vi "ReadUarmCoordinatesCompareV3.vi"(6 "error in":errorcluster, 8 "Machine In":refnum<visa-resource-name>, 9 "INPUT Z Coord":dbl, 10 "INPUT X Coord":dbl, 11 "INPUT Y Coord":dbl) -> (0 "x = y?":bool, 1 "OUTPUT Z Coord":dbl, 2 "OUTPUT X Coord":dbl, 3 "OUTPUT Y Coord":dbl, 4 "error out":errorcluster, 5 "Machine Out":refnum<visa-resource-name>)   [LabVIEW 2018]
panel:
  in  "Write Buffer":string
  out "read buffer":string="$22 ok VSwiftPro\r\n$22 ok VSwiftPro\r\n@5 V1\r\n$22 ok VSwiftPro\r\n$22 ok VSwiftPro\r\n$22 ok VSwiftPro\r\n$22 ok VSwiftPro\r\n$22 ok VSwiftPro\r\n$22 ok VSwiftPro\r\n$62 ok X157.66 Y1.93 Z-2.12\r\n$22 ok VSwiftPro\r\nstart\necho:Marlin 1.1.0-RC7\necho: Last Updatstart\necho:Marlin 1.1.0-RC7\necho: Last Updated: 2016-07-31 12:00 | Author: (none, default config)\nCompiled: Oct 25 2017\necho: Free Memory: 2376  PlannerBufferBytes: 924\necho:Hardcoded Default Settings Loaded\necho:Steps per unit:\necho:  M92 X320.00 Y320.00 Z320.00 E84.88\necho:Maximum feedrates (mm/s):\necho:  M203 X2000.00 Y2000.00 Z2000.00 E25.00\necho:Maximum Acceleration (mm/s2):\necho:  M201 X2000 Y2000 Z2000 E10000\necho:Accelerations: P=printing, R=retract and T=travel\necho:  M204 P25.00 R25.00 T100.00\necho:Advanced variables: S=Min feedrate (mm/s), T=Min travel feedrate (mm/s), B=minimum segment time (ms), X=maximum XY jerk (mm/s),  Z=maximum Z jerk (mm/s),  E=maximum E jerk (mm/s)\necho:  M205 S0.00 T0.00 B20000 X1.00 Z1.00 E5.00\necho:Home offset (mm)\necho:  M206 X0.00 Y0.00 Z0.00\necho:PID settings:\necho:  M301 P22.20 I1.08 D114.00\necho:Filament settings: Disabled\necho:  M200 D1.75\necho:  M200 D0\n"
  in  "G Code Command":string="#n P2220\n "
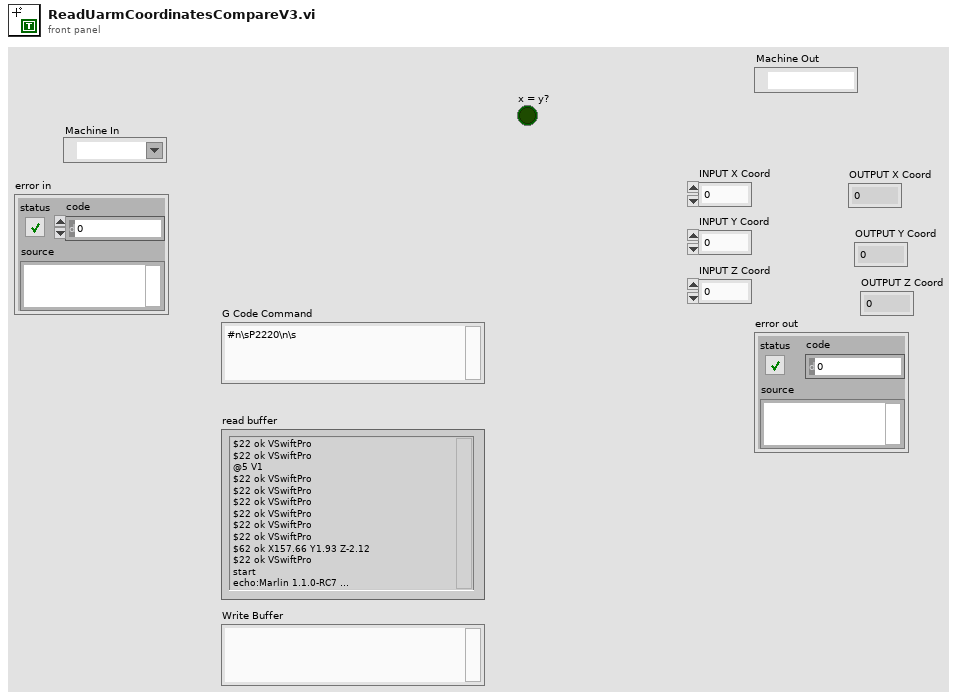
[diagram p1: front panel]
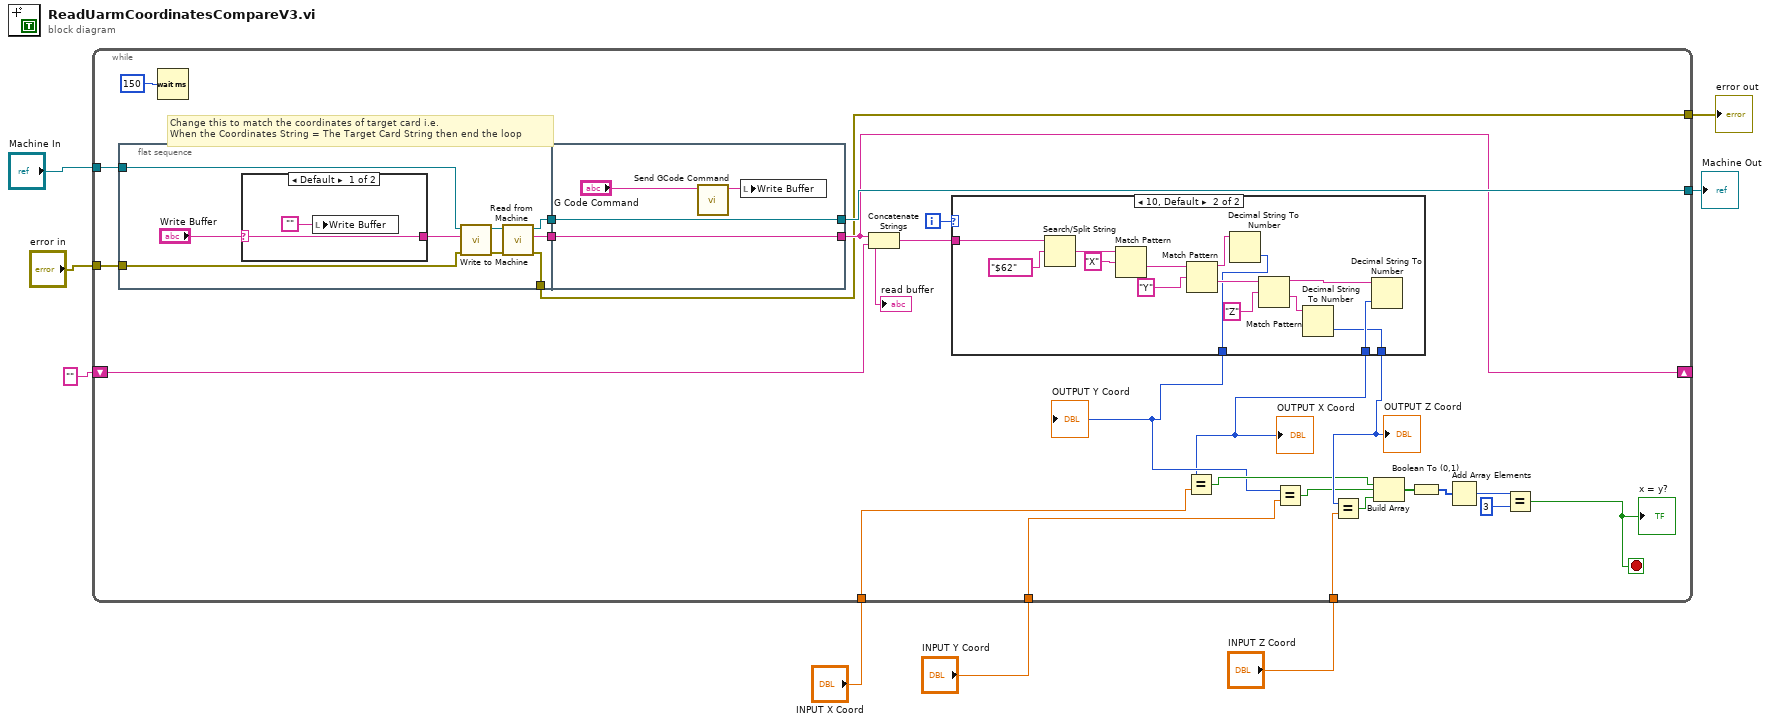
[diagram p0: block diagram]
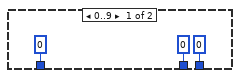
[diagram p2: hidden frame]
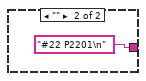
[diagram p3: hidden frame]
diagram:
  n1 = while {
    tunnel: "Machine In" -> [w32]
    tunnel: "error in" -> [w30]
    shift-right: [w26] -> _
    shift-left: "" -> [w31]
    tunnel: [w29] -> w2
    tunnel: "INPUT X Coord" -> [w23]
    tunnel: "INPUT Y Coord" -> [w22]
    tunnel: "INPUT Z Coord" -> [w20]
    tunnel: [w9] -> w1
    i -> [w24]
    stop <- w12 stop-if-true
    # "Change this to match the coordinates of target card i.e.\nWhen the Coordinates String = The Target Card String then end the loop"
    n2 = flat-sequence {
      tunnel: w32 -> [w55]
      tunnel: w30 -> [w53]
      tunnel: [w54] -> w28
      tunnel: [w52] -> w27
      tunnel: [w51] -> w9
      tunnel: [w65] -> w29
      tunnel: [w66] -> w26
      tunnel: w28 -> [w66]
      tunnel: w27 -> [w65]
      frame #0 {
        n3 = case shown="Default" "Write Buffer" {
          selector: "Write Buffer" -> [w61 _]
          tunnel: [w61 "#22 P2201\n"] -> w58
          frame Default {
            n4 = local write "Write Buffer"("") -> ()
          }
          frame "" {
          }
        }
        n5 = call "Write to Machine .vi"("error in (no error)"=w53, "G-Code String In"=w58, "Machine In"=w55) -> ("error out"=w56:errorcluster, "Machine Out"=w57:refnum<visa-resource-name>)  [unwired: 7 in]
        n6 = call "Read from Machine.vi"("error in (no error)"=w56, "Machine In"=w57) -> ("error out"=w51:errorcluster, "read buffer"=w54:string, "Machine Out"=w52:refnum<visa-resource-name>)  [unwired: 7 in]
      }
      frame #1 {
        n7 = call "Send GCode Command.vi"("G-Code Command in"="G Code Command") -> ("G-Code Command out"=w64:string)  [unwired: 10 in]
        n8 = local write "Write Buffer"(w64) -> ()
      }
    }
    n9 = Wait (ms)(milliseconds to wait=u32 150) -> ()  [unwired: 1 out]
    n10 = Concatenate Strings(w26, w31) -> (w25:string)
    "read buffer" <- w25
    n11 = case shown="10, Default" w24 {
      tunnel: w25 -> [_ w40]
      tunnel: [0 w39] -> w11
      tunnel: [0 w38] -> w10
      tunnel: [0 w37] -> w21
      frame 0..9 {
      }
      frame 10, Default {
        n12 = Search/Split String(string=w40, search string/char (-)="$62") -> (match + rest of string=w49:string)  [unwired: 1 in, 2 out]
        n13 = Match Pattern(string=w49, regular expression="X") -> (after substring=w45:string)  [unwired: 1 in, 3 out]
        n14 = Match Pattern(string=w45, regular expression="Y") -> (before substring=w44:string, after substring=w43:string)  [unwired: 1 in, 2 out]
        n15 = Decimal String To Number(string=w44) -> (number=w39:i32)  [unwired: 2 in, 1 out]
        n16 = Match Pattern(string=w43, regular expression="Z") -> (before substring=w42:string, after substring=w41:string)  [unwired: 1 in, 2 out]
        n17 = Decimal String To Number(string=w41) -> (number=w37:i32)  [unwired: 2 in, 1 out]
        n18 = Decimal String To Number(string=w42) -> (number=w38:i32)  [unwired: 2 in, 1 out]
      }
    }
    "OUTPUT Y Coord" <- w11
    "OUTPUT X Coord" <- w10
    "OUTPUT Z Coord" <- w21
    n19 = Equal?(x=w10, y=w23) -> (x = y?=w19:bool)
    n20 = Equal?(x=w11, y=w22) -> (x = y?=w18:bool)
    n21 = Equal?(x=w21, y=w20) -> (x = y?=w17:bool)
    n22 = Build Array(w19, w18, w17) -> (w16:bool[])
    n23 = Boolean To (0,1)(Boolean=w16) -> (0, 1=w15:i16[])
    n24 = Add Array Elements(numeric array=w15) -> (sum=w14:i16)
    n25 = Equal?(x=w14, y=i16 3) -> (x = y?=w12:bool)
    "x = y?" <- w12
  }
  "Machine Out" <- w2
  "error out" <- w1
